vi "Listen To Msg.vi"(7 "Actor in":refnum<class "Actor.lvclass">, 10 "Msg":refnum<class "Msg.lvclass">) -> (0 "Error out":errorcluster, 2 "Msg Output":refnum<class "Msg Output.lvclass">, 5 "Actor out":refnum<class "Actor.lvclass">)   [LabVIEW 2025, in "jettl.lvlib"]
uses:
  jettl.lvlib
  Actor/Actor.lvclass
  Msg/Msg.lvclass
  Msg Output/Msg Output.lvclass
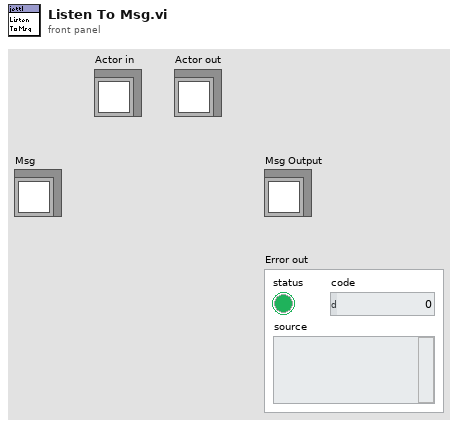
[diagram p1: front panel]
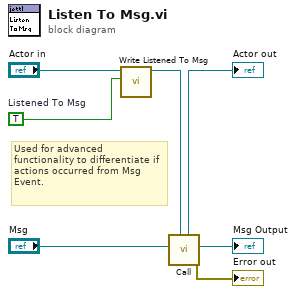
[diagram p0: block diagram]
diagram:
  w3 = TRUE  # Listened To Msg
  # "Used for advanced functionality to differentiate if actions occurred from Msg Event."
  n1 = call-dynamic "Write Listened To Msg.vi"("Listened To Msg"=w3, "Actor in"="Actor in") -> ("Actor out"=w4:refnum<class "Actor.lvclass">)  [unwired: 9 in]
  n2 = call "Call.vi"("Actor in"=w4, "Msg"="Msg") -> ("Error out"=→"Error out":errorcluster, "Msg Output"=→"Msg Output":refnum<class "Msg Output.lvclass">, "Actor out"=→"Actor out":refnum<class "Actor.lvclass">)  [unwired: 7 in]
